vi "R(T) T(t) SETP(t) with ramp332 DC ramp current(File overwrite Fixed)_1.vi"(0 "I":dbl=1e-06 min=1e-09 max=1.0 step=1e-06 format="%.4e", 1 "Ti":dbl min=0.0 max=400.0 format="%.3f", 2 "Tf":dbl=4.0 min=0.0 max=400.0 format="%.3f", 3 "Ramp":ext format="%.3f", 4 "Range":dbl=3.0 format="%.2f", 7 "Measurement":bool=TRUE, 8 "Auto\nTemp?":bool=TRUE) -> ()   [LabVIEW 2012]
panel:
  in  "write buffer":string
  out "read buffer":string
  out "VISA resource name out":refnum<visa-resource-name>
  in  "VISA resource name":refnum<visa-resource-name>
  out "?":cluster{dbl, dbl}[](graph)
  out "?":cluster{"X":dbl, "Y":dbl}[](graph)
  in  "x data precision":i16
  in  "y data precision":i16
  in  "Path":path
  in  "File name":string
  in  "Autorange":bool=TRUE
  in  "Volt Delay":u32=50
  in  "Voltmeter PLC":dbl=1.0 min=0.01 max=60.0 step=0.01 format="%.2f"
  in  "Voltage Compliance":dbl=12.0 min=0.1 max=105.0 step=0.1 format="%.2f"
  in  "minutes to wait before start":u32=5
  out "R/Ohm":dbl=1e-09 min=-1.0 step=1e-09 format="%.3e"
  out "T/K":dbl min=0.0 step=0.01 format="%.3f"
  in  "Delay time":sgl min=0 step=1 format="%.2f"
  # "ON"
  # "OFF"
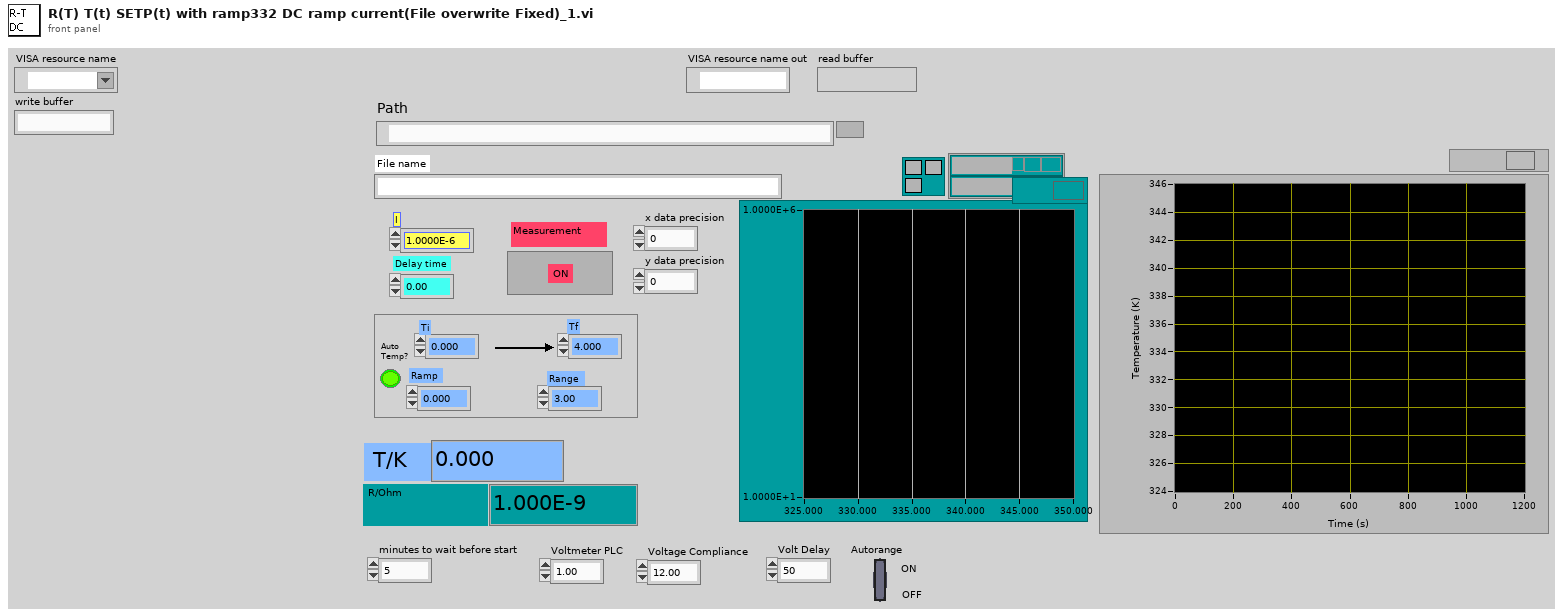
[diagram p1: front panel]
types:
  T1 = enum16{"open", "replace", "create", "open or create", "replace or create", "replace or create with confirmation"}
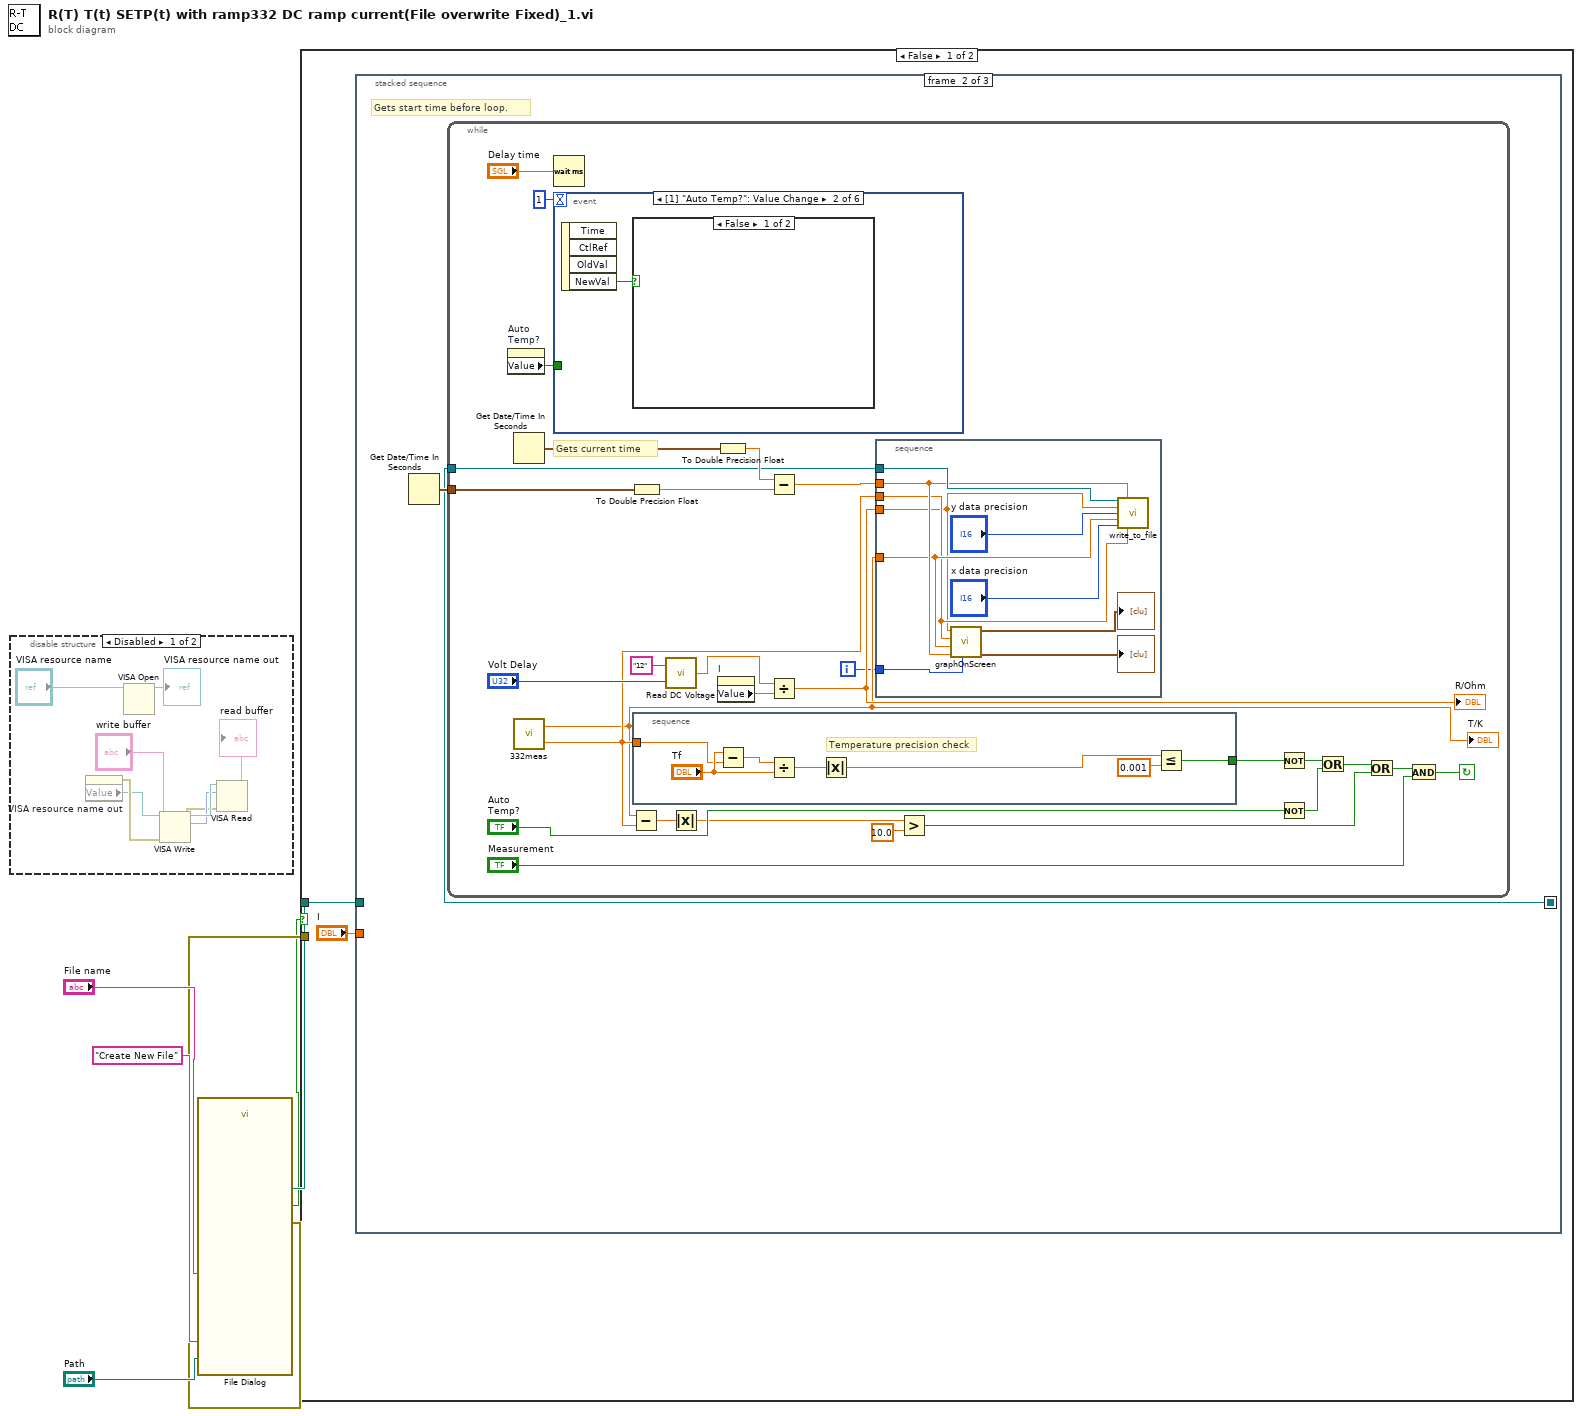
[diagram p0: block diagram]
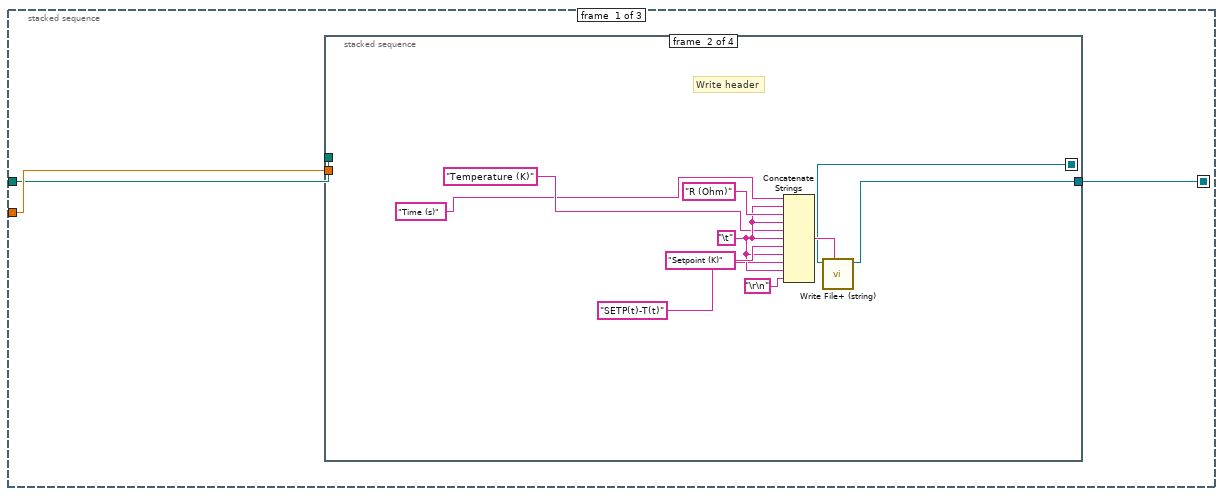
[diagram p3: hidden frame]
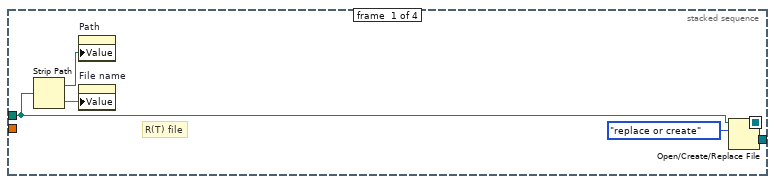
[diagram p4: hidden frame]
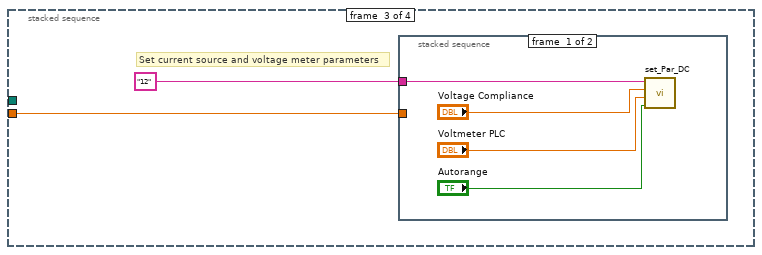
[diagram p5: hidden frame]
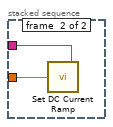
[diagram p6: hidden frame]
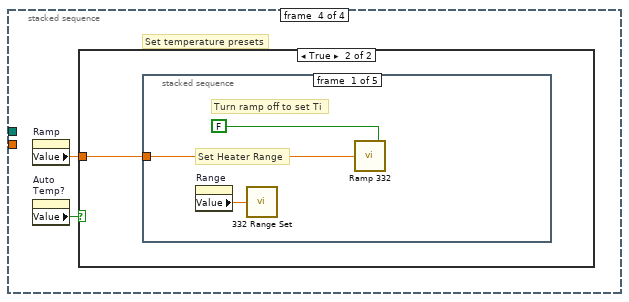
[diagram p7: hidden frame]
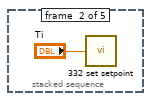
[diagram p9: hidden frame]
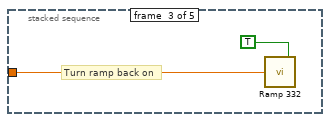
[diagram p10: hidden frame]
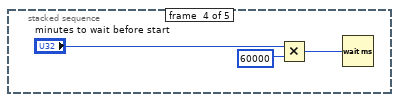
[diagram p11: hidden frame]
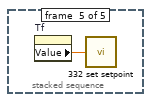
[diagram p12: hidden frame]
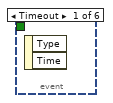
[diagram p13: hidden frame]
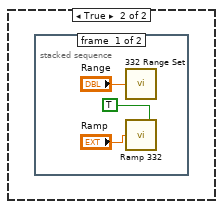
[diagram p14: hidden frame]
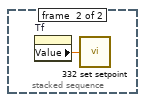
[diagram p15: hidden frame]
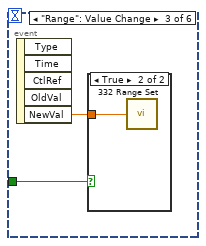
[diagram p16: hidden frame]
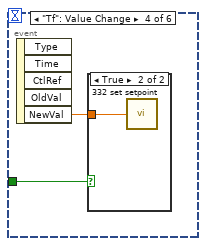
[diagram p18: hidden frame]
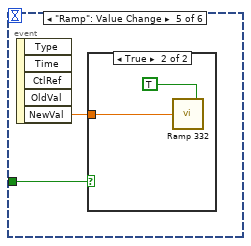
[diagram p20: hidden frame]
diagram:
  n1 = disable-structure shown="Disabled" {
    frame Disabled {
      n2 = property on="VISA resource name out" class="VISAName"() -> (error out=w13:errorcluster, "Value"=w12:refnum<visa-resource-name>)  [unwired: 2 in, 1 out]
      n3 = VISA Open(VISA resource name="VISA resource name") -> (VISA resource name=→"VISA resource name out":refnum<visa-resource-name>)  [unwired: 4 in, 1 out]
      n4 = VISA Write(VISA resource name=w12, write buffer="write buffer", error in (no error)=w13) -> (VISA resource name out=w11:refnum<visa-resource-name>, return count=w10:u32, error out=w9:errorcluster)
      n5 = VISA Read(VISA resource name=w11, byte count=w10, error in (no error)=w9) -> (read buffer=→"read buffer":string)  [unwired: 3 out]
    }
    frame Enabled {
    }
  }
  n6 = call "File Dialog"("start path"="Path", "prompt"="Create New File", "default name"="File name") -> ("selected path"=w3:path, "cancelled"=w1:bool, "error out"=w2:errorcluster)  [unwired: 9 in, 1 out]
  n7 = case shown="False" w1 {
    tunnel: w3 -> [w17 _]
    tunnel: w2 -> [_ _]
    frame False {
      n8 = stacked-sequence {
        seq-local: [w18 _ _] -> [_ w57 w124]
        tunnel: "I" -> [w20 _ w125]
        tunnel: w17 -> [w19 _ _]
        frame #0 {
          n9 = stacked-sequence {
            seq-local: [w21 _ _ _] -> [_ w34 _ _]
            tunnel: w20 -> [_ _ w36 _]
            tunnel: w19 -> [w22 _ _ _]
            tunnel: [_ w33 _ _] -> w18
            frame #0 {
              # "R(T) file"
              n10 = Strip Path(path=w22) -> (stripped path=w23:path, name=w24:string)
              n11 = property on="Path" class="Path"("Value"=w23) -> ()  [unwired: 2 in, 2 out]
              n12 = property on="File name" class="Str"("Value"=w24) -> ()  [unwired: 2 in, 2 out]
              n13 = Open/Create/Replace File(file path (use dialog)=w22, operation (0:open)=T1."replace or create") -> (refnum out=w21:refnum<file>)  [unwired: 4 in, 2 out]
            }
            frame #1 {
              w30 = "\t"
              # "Write header"
              n14 = Concatenate Strings("Time (s)" ("string"), w30, "R (Ohm)" ("string"), w30, "Temperature (K)" ("string"), w30, "Setpoint (K)" ("string"), w30, "SETP(t)-T(t)" ("string"), w30, "\r\n") -> (w35:string)
              n15 = call <vilib>:"Write File+ (string).vi"("string"=w35, "refnum"=w34) -> ("dup refnum"=w33:refnum<file>)  [unwired: 5 in, 2 out]
            }
            frame #2 {
              # "Set current source and voltage meter parameters"
              n16 = stacked-sequence {
                tunnel: "12" ("Address") -> [w41 w43]
                tunnel: w36 -> [_ w42]
                frame #0 {
                  n17 = call "set_Par_DC.vi"("Autorange"="Autorange", "Voltmeter PLC"="Voltmeter PLC", "Voltage Compliance"="Voltage Compliance", "Address"=w41) -> ()
                }
                frame #1 {
                  n18 = call "Set DC Current Ramp.vi"("Address"=w43, "Current"=w42) -> ()
                }
              }
            }
            frame #3 {
              # "Set temperature presets"
              n19 = property on="Ramp" class="DigNum (strict)"() -> ("Value"=w44:ext)  [unwired: 2 in, 2 out]
              n20 = property on="Auto\nTemp?" class="Bool (strict)"() -> ("Value"=w45:bool)  [unwired: 2 in, 2 out]
              n21 = case shown="True" w45 {
                tunnel: w44 -> [_ w46]
                frame False {
                }
                frame True {
                  n22 = stacked-sequence {
                    tunnel: w46 -> [w48 _ w52 _ _]
                    frame #0 {
                      # "Set Heater Range"
                      # "Turn ramp off to set Ti"
                      n23 = property on="Range" class="DigNum (strict)"() -> ("Value"=w47:dbl)  [unwired: 2 in, 2 out]
                      n24 = call "332 Range Set.vi"("Power Range: 93C\n0=OFF, 1=Low, 2=Med, 3=High"=w47) -> ()
                      n25 = call "Ramp 332.vi"("On"=FALSE, "K/min"=w48) -> ()
                    }
                    frame #1 {
                      n26 = call "332 set setpoint.vi"("Set Temperature SetPoint:332"="Ti") -> ()
                    }
                    frame #2 {
                      # "Turn ramp back on"
                      n27 = call "Ramp 332.vi"("On"=TRUE, "K/min"=w52) -> ()
                    }
                    frame #3 {
                      n28 = Multiply(x="minutes to wait before start", y=u32 60000) -> (x*y=w54:u32)
                      n29 = Wait (ms)(milliseconds to wait=w54) -> ()  [unwired: 1 out]
                    }
                    frame #4 {
                      n30 = property on="Tf" class="DigNum (strict)"() -> ("Value"=w56:dbl)  [unwired: 2 in, 2 out]
                      n31 = call "332 set setpoint.vi"("Set Temperature SetPoint:332"=w56) -> ()
                    }
                  }
                }
              }
            }
          }
        }
        frame #1 {
          # "Gets start time before loop."
          n32 = Get Date/Time In Seconds() -> (seconds since 1Jan1904=w58:timestamp)
          n33 = while {
            tunnel: w58 -> [w71]
            tunnel: w57 -> [w64]
            i -> [w59]
            stop <- w87 continue-if-true
            # "Gets current time"
            n34 = property on="Auto\nTemp?" class="Bool (strict)"() -> ("Value"=w83:bool)  [unwired: 2 in, 2 out]
            n35 = Get Date/Time In Seconds() -> (seconds since 1Jan1904=w73:timestamp)
            n36 = call "332meas.vi"() -> ("332 Temp [K]"=w60:dbl, "332 Temp Setpoint [K]"=w62:dbl)  [unwired: 1 in]
            "T/K" <- w60
            n37 = Wait (ms)(milliseconds to wait="Delay time") -> ()  [unwired: 1 out]
            n38 = event shown="[1] \"Auto Temp?\": Value Change" {
              selector: _ -> [_ _ _ _ _ _]
              dyn-events: _ -> [_ _ _ _ _ _]
              timeout: 1 -> [_ _ _ _ _ _]
              tunnel: w83 -> [_ _ w111 w113 w116 _]
              event Timeout {
                n39 = event-data() -> ()  [unwired: 1 in, 2 out]
              }
              event "Auto\nTemp?": Value Change {
                n40 = event-data() -> ("NewVal"=w105:bool)  [unwired: 1 in, 3 out]
                n41 = case shown="False" w105 {
                  frame False {
                  }
                  frame True {
                    n42 = stacked-sequence {
                      frame #0 {
                        n43 = call "332 Range Set.vi"("Power Range: 93C\n0=OFF, 1=Low, 2=Med, 3=High"="Range") -> ()
                        n44 = call "Ramp 332.vi"("On"=TRUE, "K/min"="Ramp") -> ()
                      }
                      frame #1 {
                        n45 = property on="Tf" class="DigNum (strict)"() -> ("Value"=w109:dbl)  [unwired: 2 in, 2 out]
                        n46 = call "332 set setpoint.vi"("Set Temperature SetPoint:332"=w109) -> ()
                      }
                    }
                  }
                }
              }
              event "Range": Value Change {
                n47 = event-data() -> ("NewVal"=w110:dbl)  [unwired: 1 in, 4 out]
                n48 = case shown="True" w111 {
                  tunnel: w110 -> [_ w112]
                  frame False {
                  }
                  frame True {
                    n49 = call "332 Range Set.vi"("Power Range: 93C\n0=OFF, 1=Low, 2=Med, 3=High"=w112) -> ()
                  }
                }
              }
              event "Tf": Value Change {
                n50 = event-data() -> ("NewVal"=w114:dbl)  [unwired: 1 in, 4 out]
                n51 = case shown="True" w113 {
                  tunnel: w114 -> [_ w115]
                  frame False {
                  }
                  frame True {
                    n52 = call "332 set setpoint.vi"("Set Temperature SetPoint:332"=w115) -> ()
                  }
                }
              }
              event "Ramp": Value Change {
                n53 = event-data() -> ("NewVal"=w117:ext)  [unwired: 1 in, 4 out]
                n54 = case shown="True" w116 {
                  tunnel: w117 -> [_ w118]
                  frame False {
                  }
                  frame True {
                    n55 = call "Ramp 332.vi"("On"=TRUE, "K/min"=w118) -> ()
                  }
                }
              }
              event "I": Value Change {
                n56 = event-data() -> ("NewVal"=w120:dbl)  [unwired: 1 in, 4 out]
                n57 = stacked-sequence {
                  tunnel: w120 -> [_ w122]
                  frame #0 {
                    # "Wait until measurement\nfinished"
                    n58 = Wait (ms)(milliseconds to wait=u32 1000) -> ()  [unwired: 1 out]
                  }
                  frame #1 {
                    n59 = call "Set DC Current.vi"("Address"="24" ("address string"), "Current"=w122) -> ()
                  }
                }
              }
            }
            n60 = Subtract(x=w60, y=w62) -> (x-y=w70:dbl)
            n61 = To Double Precision Float(number=w71) -> (double precision float=w72:dbl)
            n62 = stacked-sequence {
              tunnel: [w99] -> w86
              tunnel: w62 -> [w98]
              frame #0 {
                # "Temperature precision check"
                n63 = Subtract(x="Tf", y=w98) -> (x-y=w102:dbl)
                n64 = Divide(x=w102, y="Tf") -> (x/y=w103:dbl)
                n65 = Absolute Value(x=w103) -> (abs(x)=w101:dbl)
                n66 = Less Or Equal?(x=w101, y=0.001) -> (x <= y?=w99:bool)
              }
            }
            n67 = call "Read DC Voltage.vi"("Volt Delay"="Volt Delay", "Address"="12" ("address string")) -> ("Voltage"=w76:dbl)
            n68 = Absolute Value(x=w70) -> (abs(x)=w66:dbl)
            n69 = To Double Precision Float(number=w73) -> (double precision float=w74:dbl)
            n70 = property on="I" class="DigNum (strict)"() -> ("Value"=w77:dbl)  [unwired: 2 in, 2 out]
            n71 = Subtract(x=w74, y=w72) -> (x-y=w61:dbl)
            n72 = Divide(x=w76, y=w77) -> (x/y=w63:dbl)
            "R/Ohm" <- w63
            n73 = stacked-sequence {
              tunnel: w64 -> [w97]
              tunnel: w63 -> [w88]
              tunnel: w62 -> [w89]
              tunnel: w61 -> [w91]
              tunnel: w60 -> [w90]
              tunnel: w59 -> [w92]
              frame #0 {
                n74 = call "graphOnScreen.vi"("Connect to loop iteration"=w92, "Time"=w91, "332 Temp [K]"=w90, "332 Temp Setpoint [K]"=w89, "R(ohm)"=w88) -> ("T(t)"=→"?":cluster{"X":dbl, "Y":dbl}[], 3:→"?":cluster{dbl, dbl}[])  [unwired: 5 in]
                n75 = call "write_to_file.vi"("refnum"=w97, "Time"=w91, "y data"=w88, "y data precision"="y data precision", "x data"=w90, "x data precision"="x data precision", "Setpoint"=w89) -> ()  [unwired: 8 in, 1 out]
              }
            }
            n76 = Greater?(x=w66, y=10.0) -> (0:w65:bool)
            n77 = Not(x=w86) -> (.not. x?=w84:bool)
            n78 = Not(x="Auto\nTemp?") -> (.not. x?=w79:bool)
            n79 = Or(x=w84, y=w79) -> (x .or. y?=w69:bool)
            n80 = Or(x=w69, y=w65) -> (x .or. y?=w68:bool)
            n81 = And(x=w68, y="Measurement") -> (x .and. y?=w87:bool)
          }
        }
        frame #2 {
          w126 = "12" ("Address")
          n82 = call "Send to Volt Meter.vi"("Address"=w126, "Data"=":trig:sour imm;:init") -> ()
          n83 = stacked-sequence {
            tunnel: w126 -> [w129 w130]
            tunnel: w125 -> [w128 _]
            frame #0 {
              n84 = call "Set DC Current Ramp to Zero.vi"("Address"=w129, "Current"=w128) -> ()
            }
            frame #1 {
              n85 = call "disarm.vi"("address string"=w130) -> ()  [unwired: 1 in, 1 out]
            }
          }
          n86 = Close File(refnum=w124) -> ()  [unwired: 1 in, 2 out]
        }
      }
    }
    frame True {
    }
  }
